vi "子界面-查看某框-不显示界面-只读穿透图模式.vi"(0 "框号":dbl format="%#_13g", 1 "框组":T3(array[cluster]), 2 "临界Z值":i32, 4 "临界面积百分比值":dbl, 5 "预先配置的灰度阈值":dbl, 6 "穿透图原始路径":path, 7 "部位信息":string[](array[string])=["", "34.500000", "32.500000", "1121", "34", "54.955926", "分层类", "不合格", ""], 12 "产品规格":cluster{"产品长度（周长）（mm）":dbl, "产品宽度（母线长）（mm）":dbl}) -> (14 "弥散类检测结果":string[][](table), 19 "分层类检测结果":string[][](table))   [LabVIEW 2018]
uses:
  <vilib>/vision/NI_Vision_Development_Module.lvlib
panel:
  in  "Tab Control":T1
  out "?":T2(plugin-control)
  out "Threshold Image":T2(plugin-control)
  out "Threshold Image":T2(plugin-control)
  in  "格式字符串 3":string="%f"
  in  "分隔符（'\\'代码显示） 2":string="\t"
  out "弥散和分层临界灰度值":i64
  out "弥散缺陷个数":i32
  out "分层缺陷个数":i32
  out "合格？ 弥散类":string="fencengThreshold"
  out "合格？分层类":string="fencengThreshold"
  out "弥散测量结果":dbl[][](array[numeric]) format="%.2f"
  out "面积 (pixels)":i32
  in  "格式字符串 2":string="%f"
  in  "分隔符（'\\'代码显示）":string="\t"
  out "分层测量结果":dbl[][](array[numeric]) format="%.2f"
  out "缺陷初步分类的临界值":sgl format="%#.3f"
  # "所选区域信息"
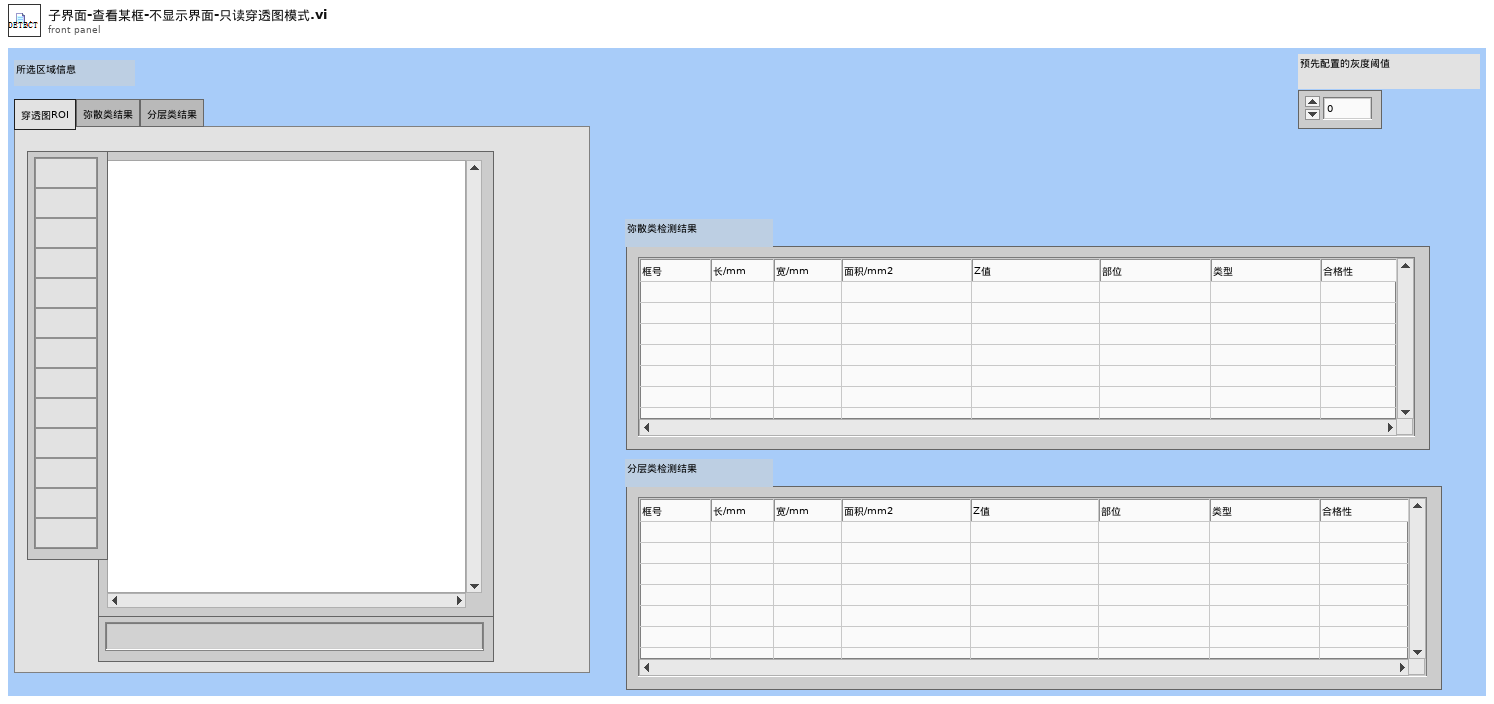
[diagram p1: front panel]
types:
  T1 = typedef "控件2.ctl" = enum32{"穿透图ROI", "弥散类结果", "分层类结果"}
  T2 = typedef "IMAQ Image.ctl" = refnum<image>
  T3 = cluster{"Global Rectangle":i32[], "Contours":cluster{"Contour Type":u32, "ROI Type":u32, "Points":i32[]}[]}[]
  T4 = typedef "Image Type" = u32
  T5 = typedef "Particle Parameters" = i32
  T6 = cluster{"Measurement Parameter":T5, "Range Lower Value":dbl, "Range Upper Value":dbl, "Range":bool, "Measurement Type":bool}[]
  T7 = cluster{"Global Rectangle":i32[], "Contours":cluster{"Contour Type":u32, "ROI Type":u32, "Points":i32[]}[]}
  T8 = cluster{"histogram":u32[], "Minimal Value":sgl, "Maximal Value":sgl, "Starting Value":sgl, "Interval Width":sgl, "Mean Value":sgl, "Standard  Variation":sgl, "Area (pixels)":i32}
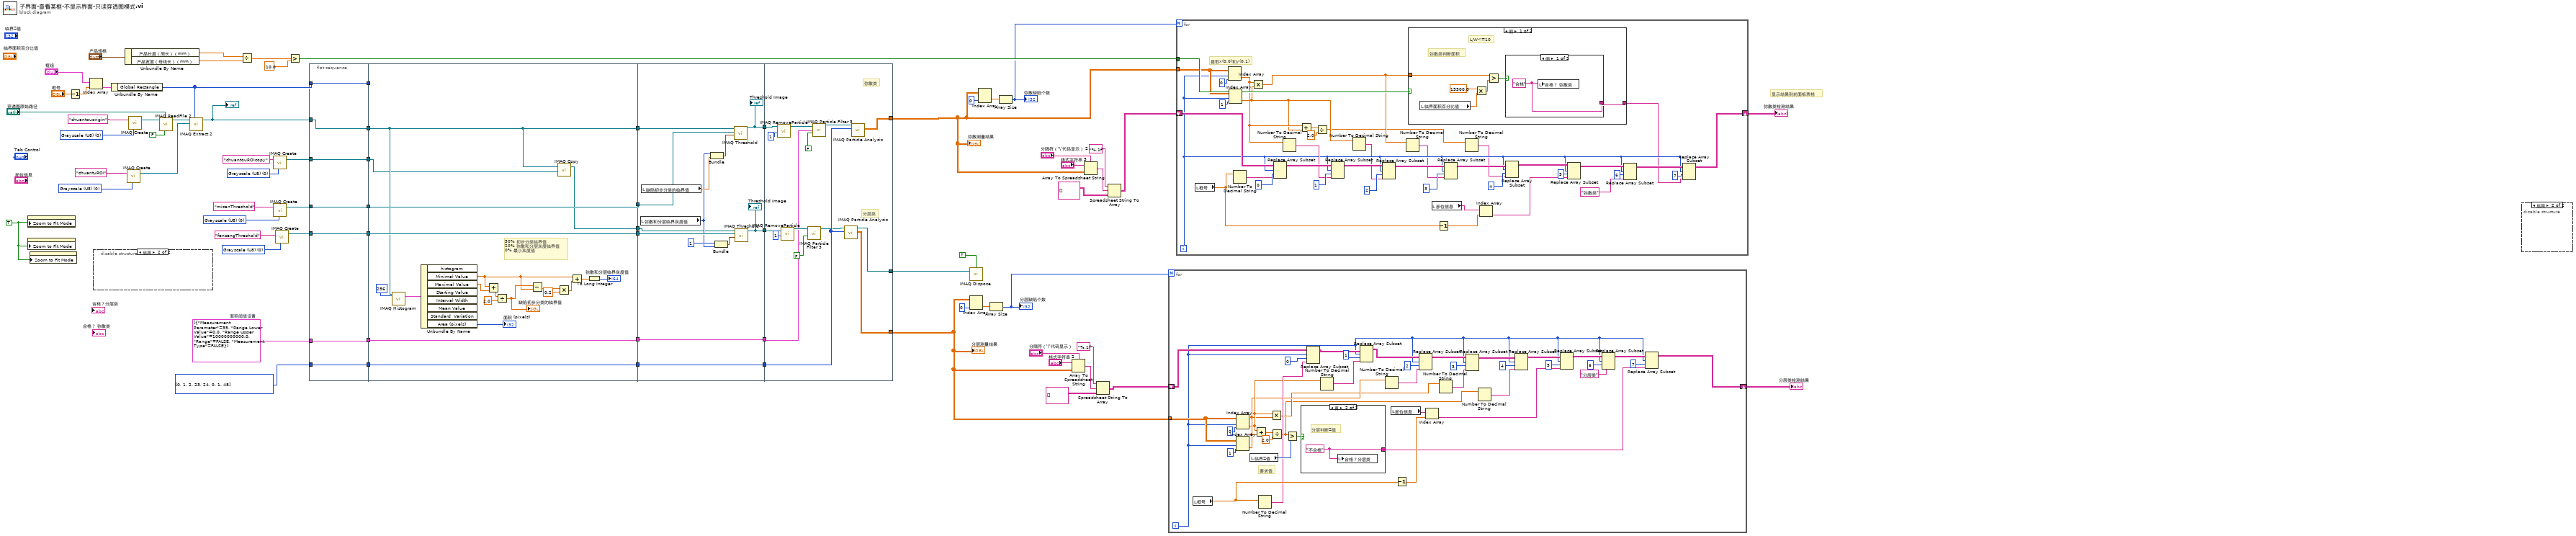
[diagram p0: block diagram]
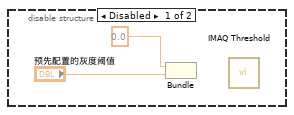
[diagram p2: hidden frame]
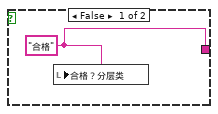
[diagram p3: hidden frame]
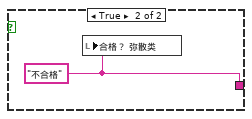
[diagram p4: hidden frame]
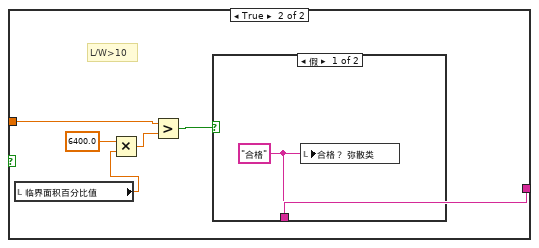
[diagram p5: hidden frame]
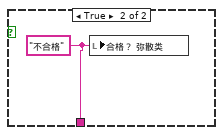
[diagram p6: hidden frame]
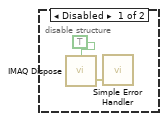
[diagram p7: hidden frame]
diagram:
  w1 = T4 0 items=["Grayscale (U8)", "Grayscale (I16)", "Grayscale (SGL)", "Complex (CSG)", "RGB (U32)", "HSL (U32)", "RGB (U64)", "Grayscale (U16)"] ("Image Type")
  w6 = TRUE ("Zoom to Fit Mode")
  w51 = T4 0 items=["Grayscale (U8)", "Grayscale (I16)", "Grayscale (SGL)", "Complex (CSG)", "RGB (U32)", "HSL (U32)", "RGB (U64)", "Grayscale (U16)"] ("Image Type")
  w52 = T4 0 items=["Grayscale (U8)", "Grayscale (I16)", "Grayscale (SGL)", "Complex (CSG)", "RGB (U32)", "HSL (U32)", "RGB (U64)", "Grayscale (U16)"] ("Image Type")
  w55 = T4 0 items=["Grayscale (U8)", "Grayscale (I16)", "Grayscale (SGL)", "Complex (CSG)", "RGB (U32)", "HSL (U32)", "RGB (U64)", "Grayscale (U16)"] ("Image Type")
  w29 = i32[] [0, 1, 2, 23, 24, 0, 1, 48] items=["Bounding Rect Width", "Bounding Rect Height"] ("Pixel Measurements")
  w33 = T6 [{"Measurement Parameter"=35, "Range Lower Value"=0.0, "Range Upper Value"=10000000000.0, "Range"=FALSE, "Measurement Type"=FALSE}]  # 面积阈值设置
  w69 = T4 0 items=["Grayscale (U8)", "Grayscale (I16)", "Grayscale (SGL)", "Complex (CSG)", "RGB (U32)", "HSL (U32)", "RGB (U64)", "Grayscale (U16)"] ("Image Type")
  # "显示结果到前面板表格"
  n1 = property class="ImageControl"("Zoom to Fit Mode"=w6) -> ()  [unwired: 2 in, 2 out]
  n2 = property class="ImageControl"("Zoom to Fit Mode"=w6) -> ()  [unwired: 2 in, 2 out]
  n3 = property class="ImageControl"("Zoom to Fit Mode"=w6) -> ()  [unwired: 2 in, 2 out]
  n4 = Decrement(x="框号") -> (x-1=w71:dbl)
  n5 = Index Array(array="框组", index=w71) -> (element=w72:T7)
  n6 = disable-structure shown="启用" {
    frame Disabled {
      n7 = Bundle(0.0, "预先配置的灰度阈值"="预先配置的灰度阈值") -> ()  [unwired: 1 in, 1 out]
      n8 = call "IMAQ Threshold"() -> ()  [unwired: 6 in, 6 out]
    }
    frame Enabled {
    }
  }
  n9 = Unbundle By Name(w72) -> ("Global Rectangle"=w45:i32[])
  n10 = Unbundle By Name("产品规格") -> ("产品长度（周长）（mm）"=w63:dbl, "产品宽度（母线长）（mm）"=w62:dbl)
  n11 = call "IMAQ Create"("Image Name"="chuantuROI", "Image Type"=w55) -> ("New Image"=w54:T2)  [unwired: 3 in, 1 out]
  n12 = call "IMAQ Create"("Image Name"="chuantouorigin", "Image Type"=w69) -> ("New Image"=w57:T2)  [unwired: 3 in, 1 out]
  n13 = call "IMAQ ReadFile 2"("Use File Path Image Type"=FALSE, "File Path"="穿透图原始路径", "Image"=w57) -> ("Image Out"=w58:T2)  [unwired: 4 in, 4 out]
  n14 = call "IMAQ Extract 2"("Optional Rectangle"=w45, "Image Dst"=w54, "Image Src"=w58) -> ("Image Dst Out"=w9:T2)  [unwired: 7 in, 1 out]
  "?" <- w9
  n15 = Divide(x=w63, y=w62) -> (x/y=w66:dbl)
  n16 = call "IMAQ Create"("Image Name"="chuantouROIcopy", "Image Type"=w1) -> ("New Image"=w4:T2)  [unwired: 3 in, 1 out]
  n17 = call "IMAQ Create"("Image Name"="misanThreshold", "Image Type"=w51) -> ("New Image"=w41:T2)  [unwired: 3 in, 1 out]
  n18 = call "IMAQ Create"("Image Name"="fencengThreshold", "Image Type"=w52) -> ("New Image"=w39:T2)  [unwired: 3 in, 1 out]
  n19 = Greater?(x=w66, y=10.0) -> (0:w61:bool)
  n20 = flat-sequence {
    tunnel: w45 -> [w83]
    tunnel: w9 -> [w78]
    tunnel: [w83] -> w44
    tunnel: w41 -> [w82]
    tunnel: [w82] -> w42
    tunnel: [w81] -> w40
    tunnel: w39 -> [w81]
    tunnel: [w80] -> w34
    tunnel: w33 -> [w80]
    tunnel: [w79] -> w30
    tunnel: w29 -> [w79]
    tunnel: [w78] -> w7
    tunnel: w4 -> [w77]
    tunnel: [w77] -> w3
    tunnel: [w103] -> w43
    tunnel: [w102] -> w38
    tunnel: [w97] -> w32
    tunnel: [w96] -> w28
    tunnel: w30 -> [w96]
    tunnel: w34 -> [w97]
    tunnel: w40 -> [w102]
    tunnel: w42 -> [w103]
    tunnel: w44 -> [_]
    tunnel: [w86] -> w8
    tunnel: w7 -> [w86]
    tunnel: [w85] -> w5
    tunnel: w3 -> [w84]
    tunnel: w43 -> [w116]
    tunnel: w38 -> [w115]
    tunnel: [w105] -> w36
    tunnel: [w106] -> w35
    tunnel: w32 -> [w114]
    tunnel: [w114] -> w31
    tunnel: w28 -> [w113]
    tunnel: [w113] -> w27
    tunnel: w8 -> [w107]
    tunnel: w5 -> [w104]
    tunnel: [w117] -> w12
    tunnel: [w125] -> w20
    tunnel: [w124] -> w37
    tunnel: w36 -> [w123]
    tunnel: w35 -> [w122]
    tunnel: w31 -> [w121]
    tunnel: w27 -> [w120]
    frame #0 {
    }
    frame #1 {
      # "50% 初步分类临界值\n20% 弥散和分层灰度临界值\n0% 最小灰度值"
      n21 = call "IMAQ Histogram"("Number of Classes"=256, "Image"=w86) -> ("Histogram Report"=w100:T8)  [unwired: 8 in, 1 out]
      n22 = Unbundle By Name(w100) -> ("Minimal Value"=w88:sgl, "Maximal Value"=w94:sgl, "Area (pixels)"=→"面积 (pixels)":i32)  [unwired: 5 out]
      n23 = Add(x=w88, y=w94) -> (x+y=w93:sgl)
      n24 = Divide(x=w93, y=sgl 2.0) -> (x/y=w92:sgl)
      "缺陷初步分类的临界值" <- w92
      n25 = Subtract(x=w92, y=w88) -> (x-y=w90:sgl)
      n26 = Multiply(x=w90, y=0.2) -> (x*y=w89:dbl)
      n27 = call "IMAQ Copy"("Image Dst"=w84, "Image Src"=w86) -> ("Image Dst Out"=w85:T2)  [unwired: 4 in, 1 out]
      n28 = Add(x=w88, y=w89) -> (x+y=w87:dbl)
      n29 = To Long Integer(number=w87) -> (32bit integer=→"弥散和分层临界灰度值":i32)
    }
    frame #2 {
      n30 = local read "弥散和分层临界灰度值"() -> (w109:i64)
      n31 = local read "缺陷初步分类的临界值"() -> (w111:sgl)
      n32 = Bundle("弥散和分层临界灰度值"=w109, "缺陷初步分类的临界值"=w111) -> (w112:cluster{"弥散和分层临界灰度值":i64, "缺陷初步分类的临界值":sgl})  [unwired: 1 in]
      n33 = Bundle(1, "弥散和分层临界灰度值"=w109) -> (w108:cluster{i32, "弥散和分层临界灰度值":i64})  [unwired: 1 in]
      n34 = call "IMAQ Threshold"("Range"=w112, "Image Dst"=w116, "Image Src"=w107) -> ("Image Dst Out"=w106:T2)  [unwired: 3 in, 5 out]
      "Threshold Image" <- w106
      n35 = call "IMAQ Threshold"("Range"=w108, "Image Dst"=w115, "Image Src"=w104) -> ("Image Dst Out"=w105:T2)  [unwired: 3 in, 5 out]
      "Threshold Image" <- w105
    }
    frame #3 {
      # "分层类"
      # "弥散类"
      n36 = call "IMAQ RemoveParticle"("Number of Erosion"=1, "Image Src"=w122) -> ("Image Dst Out"=w131:T2)  [unwired: 8 in, 1 out]
      n37 = call "IMAQ RemoveParticle"("Number of Erosion"=1, "Image Src"=w123) -> ("Image Dst Out"=w128:T2)  [unwired: 8 in, 1 out]
      n38 = call "IMAQ Particle Filter 3"("Image Src"=w128, "Keep/Remove Particles (F)"=FALSE) -> ("Image Dst Out"=w118:T2)  [unwired: 11 in, 2 out]
      n39 = call "IMAQ Particle Filter 3"("Image Src"=w131, "Selection Values"=w121, "Keep/Remove Particles (F)"=FALSE) -> ("Image Dst Out"=w119:T2)  [unwired: 10 in, 2 out]
      n40 = call "IMAQ Particle Analysis"("Pixel Measurements"=w120, "Image"=w118) -> ("Particle Measurements (Pixels)"=w125:dbl[][], "Image Out (duplicate)"=w124:T2)  [unwired: 4 in, 4 out]
      n41 = call "IMAQ Particle Analysis"("Pixel Measurements"=w120, "Image"=w119) -> ("Particle Measurements (Pixels)"=w117:dbl[][])  [unwired: 4 in, 5 out]
    }
  }
  n42 = call "IMAQ Dispose"("All Images? (No)"=TRUE, "Image"=w37) -> ()  [unwired: 4 in, 1 out]
  n43 = Index Array(array=w20, index (col)=0 ("禁用的索引 (列)")) -> (element=w49:dbl[])  [unwired: 1 in]
  n44 = Index Array(array=w12, index (col)=0 ("禁用的索引 (列)")) -> (element=w47:dbl[])  [unwired: 1 in]
  n45 = Array Size(array=w49) -> (size(s)=w26:i32)
  "分层缺陷个数" <- w26
  n46 = Array Size(array=w47) -> (size(s)=w60:i32)
  "弥散缺陷个数" <- w60
  n47 = Array To Spreadsheet String(delimiter (Tab)="分隔符（'\\'代码显示）", array=w20, 3:"格式字符串 2") -> (spreadsheet string=w23:string)
  n48 = Array To Spreadsheet String(delimiter (Tab)="分隔符（'\\'代码显示） 2", array=w12, 3:"格式字符串 3") -> (spreadsheet string=w15:string)
  n49 = Spreadsheet String To Array(format string="%.1f", spreadsheet string=w23, array type (2D Dbl)=string[][] [] ("Array")) -> (array=w19:string[][])  [unwired: 1 in]
  n50 = Spreadsheet String To Array(format string="%.1f", spreadsheet string=w15, array type (2D Dbl)=string[][] [] ("Array")) -> (array=w11:string[][])  [unwired: 1 in]
  n51 = for {
    N: w26 -> [_]
    tunnel: w20 -> [w163]
    shift-right: [w141] -> w18
    shift-left: w19 -> [w152]
    i -> [w136]
    # "要求值"
    n52 = local read "框号"() -> (w161:dbl)
    n53 = Index Array(array=w163, index (row)=w136, index (col)=0 ("禁用的索引 (列)")) -> (element=w140:dbl)
    n54 = Index Array(array=w163, index (row)=w136, index (col)=1 ("禁用的索引 (列)")) -> (element=w139:dbl)
    n55 = local read "临界Z值"() -> (w169:i32)
    n56 = Add(x=w140, y=w139) -> (x+y=w170:dbl)
    n57 = Number To Decimal String(number=w161) -> (decimal integer string=w153:string)  [unwired: 1 in]
    n58 = Multiply(x=w140, y=w139) -> (x*y=w138:dbl)
    n59 = Divide(x=w170, y=2.0) -> (x/y=w135:dbl)
    n60 = Greater?(x=w135, y=w169) -> (0:w171:bool)
    n61 = case shown="真" w171 {
      tunnel: [w172 w173] -> w132
      frame False {
        w172 = "合格" ("合格？")
        n62 = local write "合格？分层类"(w172) -> ()
      }
      frame True {
        w173 = "不合格" ("合格？")
        # "分层判断Z值"
        n63 = local write "合格？分层类"(w173) -> ()
      }
    }
    n64 = Replace Array Subset(array=w152, new element=w153, index (row)=w136, index (col)=0 ("索引 (列)")) -> (w151:string[][])
    n65 = Number To Decimal String(number=w140) -> (decimal integer string=w150:string)  [unwired: 1 in]
    n66 = Replace Array Subset(array=w151, new element=w150, index (row)=w136, index (col)=1 ("索引 (列)")) -> (w148:string[][])
    n67 = Number To Decimal String(number=w139) -> (decimal integer string=w149:string)  [unwired: 1 in]
    n68 = local read "部位信息"() -> (w165:string[])
    n69 = Decrement(x=w161) -> (x-1=w164:dbl)
    n70 = Replace Array Subset(array=w148, new element=w149, index (row)=w136, index (col)=2 ("索引 (列)")) -> (w147:string[][])
    n71 = Index Array(array=w165, index=w164) -> (element=w134:string)
    n72 = Number To Decimal String(number=w138) -> (decimal integer string=w146:string)  [unwired: 1 in]
    n73 = Replace Array Subset(array=w147, new element=w146, index (row)=w136, index (col)=3 ("索引 (列)")) -> (w145:string[][])
    n74 = Number To Decimal String(number=w135) -> (decimal integer string=w137:string)  [unwired: 1 in]
    n75 = Replace Array Subset(array=w145, new element=w137, index (row)=w136, index (col)=4 ("索引 (列)")) -> (w144:string[][])
    n76 = Replace Array Subset(array=w144, new element=w134, index (row)=w136, index (col)=5 ("索引 (列)")) -> (w143:string[][])
    n77 = Replace Array Subset(array=w143, new element="分层类" ("新元素/子数组"), index (row)=w136, index (col)=6 ("索引 (列)")) -> (w142:string[][])
    n78 = Replace Array Subset(array=w142, new element=w132, index (row)=w136, index (col)=7 ("索引 (列)")) -> (w141:string[][])
  }
  "分层类检测结果" <- w18
  n79 = for {
    N: w60 -> [_]
    tunnel: w61 -> [w212]
    tunnel: w12 -> [w211]
    shift-right: [w191] -> w10
    shift-left: w11 -> [w199]
    i -> [w189]
    # "提取x(0,0)和y(0,1)"
    n80 = local read "框号"() -> (w177:dbl)
    n81 = Index Array(array=w211, index (row)=w189, index (col)=0 ("禁用的索引 (列)")) -> (element=w183:dbl)
    n82 = Index Array(array=w211, index (row)=w189, index (col)=1 ("禁用的索引 (列)")) -> (element=w182:dbl)
    n83 = Number To Decimal String(number=w177) -> (decimal integer string=w200:string)  [unwired: 1 in]
    n84 = Multiply(x=w183, y=w182) -> (x*y=w187:dbl)
    n85 = Replace Array Subset(array=w199, new element=w200, index (row)=w189, index (col)=0 ("索引 (列)")) -> (w198:string[][])
    n86 = Number To Decimal String(number=w183) -> (decimal integer string=w190:string)  [unwired: 1 in]
    n87 = Add(x=w183, y=w182) -> (x+y=w185:dbl)
    n88 = Divide(x=w185, y=2.0) -> (x/y=w181:dbl)
    n89 = Replace Array Subset(array=w198, new element=w190, index (row)=w189, index (col)=1 ("索引 (列)")) -> (w197:string[][])
    n90 = Number To Decimal String(number=w182) -> (decimal integer string=w188:string)  [unwired: 1 in]
    n91 = Replace Array Subset(array=w197, new element=w188, index (row)=w189, index (col)=2 ("索引 (列)")) -> (w196:string[][])
    n92 = Number To Decimal String(number=w187) -> (decimal integer string=w186:string)  [unwired: 1 in]
    n93 = case shown="假" w212 {
      tunnel: w187 -> [w218 w226]
      tunnel: [w216 w224] -> w174
      frame False {
        # "弥散类判断面积"
        # "L/W<=10"
        n94 = local read "临界面积百分比值"() -> (w214:dbl)
        n95 = Multiply(x=15500.0, y=w214) -> (x*y=w213:dbl)
        n96 = Greater?(x=w218, y=w213) -> (0:w217:bool)
        n97 = case shown="假" w217 {
          tunnel: [w219 w220] -> w216
          frame False {
            w219 = "合格" ("合格？")
            n98 = local write "合格？ 弥散类"(w219) -> ()
          }
          frame True {
            w220 = "不合格" ("合格？")
            n99 = local write "合格？ 弥散类"(w220) -> ()
          }
        }
      }
      frame True {
        # "L/W>10"
        n100 = local read "临界面积百分比值"() -> (w221:dbl)
        n101 = Multiply(x=6400.0, y=w221) -> (x*y=w223:dbl)
        n102 = Greater?(x=w226, y=w223) -> (0:w225:bool)
        n103 = case shown="假" w225 {
          tunnel: [w227 w228] -> w224
          frame False {
            w227 = "合格" ("合格？")
            n104 = local write "合格？ 弥散类"(w227) -> ()
          }
          frame True {
            w228 = "不合格" ("合格？")
            n105 = local write "合格？ 弥散类"(w228) -> ()
          }
        }
      }
    }
    n106 = local read "部位信息"() -> (w179:string[])
    n107 = Decrement(x=w177) -> (x-1=w178:dbl)
    n108 = Replace Array Subset(array=w196, new element=w186, index (row)=w189, index (col)=3 ("索引 (列)")) -> (w195:string[][])
    n109 = Number To Decimal String(number=w181) -> (decimal integer string=w180:string)  [unwired: 1 in]
    n110 = Index Array(array=w179, index=w178) -> (element=w176:string)
    n111 = Replace Array Subset(array=w195, new element=w180, index (row)=w189, index (col)=4 ("索引 (列)")) -> (w194:string[][])
    n112 = Replace Array Subset(array=w194, new element=w176, index (row)=w189, index (col)=5 ("索引 (列)")) -> (w193:string[][])
    n113 = Replace Array Subset(array=w193, new element="弥散类" ("新元素/子数组"), index (row)=w189, index (col)=6 ("索引 (列)")) -> (w192:string[][])
    n114 = Replace Array Subset(array=w192, new element=w174, index (row)=w189, index (col)=7 ("索引 (列)")) -> (w191:string[][])
  }
  "弥散类检测结果" <- w10
  n115 = disable-structure shown="启用" {
    frame Disabled {
      n116 = call "IMAQ Dispose"("All Images? (No)"=TRUE) -> ("error out"=w230:errorcluster)  [unwired: 5 in]
      n117 = call <vilib>:"Simple Error Handler.vi"("error in (no error)"=w230) -> ()  [unwired: 4 in, 5 out]
    }
    frame Enabled {
    }
  }
  "分层测量结果" <- w20
  "弥散测量结果" <- w12
